vi "Acquire Image.vi"(8 "error in (no error)":errorcluster, 9 "Cluster":T2={"Gamma::Value"=1.6, "Gain::Value"=50, "Sharpness::Value"=0, "Contrast::Value"=0.5, "Exposure::Value"=0.0078125} {"Exposure::Value" min=0.000244140625 max=0.5; "Contrast::Value" min=0.0 max=1.0; "Sharpness::Value" min=0 max=2 step=1; "Gain::Value" min=0 max=100 step=1; "Gamma::Value" min=0.01 max=10.0}, 10 "Stop":bool, 11 "QR Code Reader in":refnum<class "QR Code Reader.lvclass">) -> (0 "error out":errorcluster, 2 "Image Out":T1(plugin-control), 3 "QR Code Reader out":refnum<class "QR Code Reader.lvclass">)   [LabVIEW 2021, in "QR Code Reader.lvclass"]
uses:
  QR Code Reader.lvclass
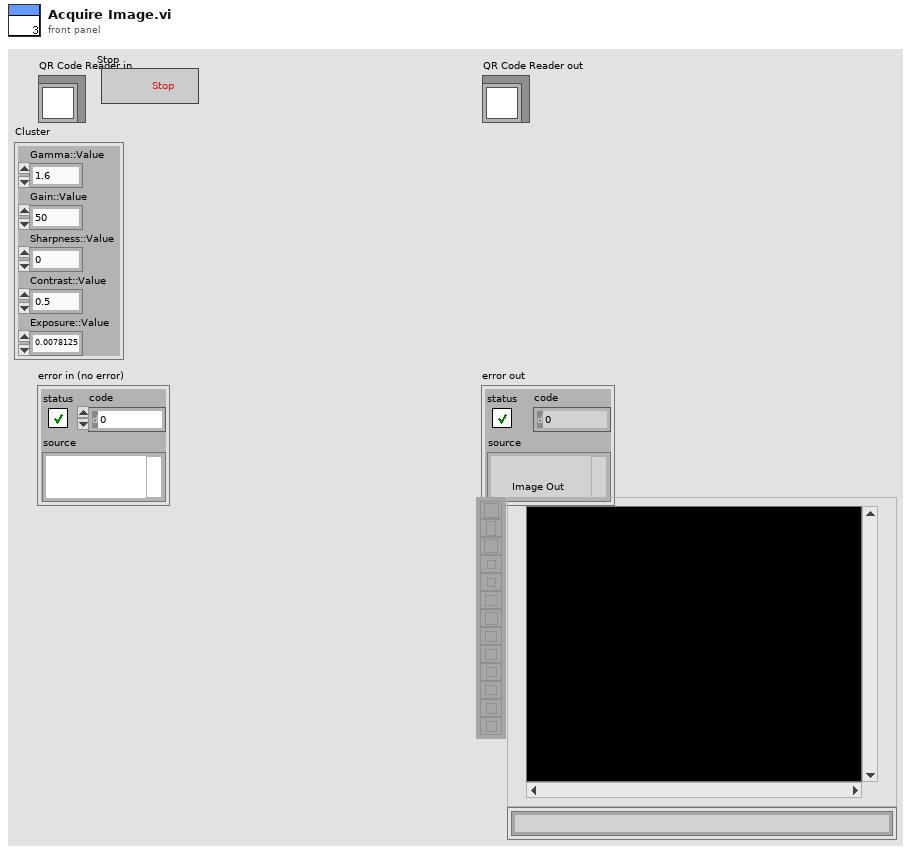
[diagram p1: front panel]
types:
  T1 = typedef "IMAQ Image.ctl" = refnum<image>
  T2 = cluster{"Gamma::Value":dbl, "Gain::Value":i64, "Sharpness::Value":i64, "Contrast::Value":dbl, "Exposure::Value":dbl}
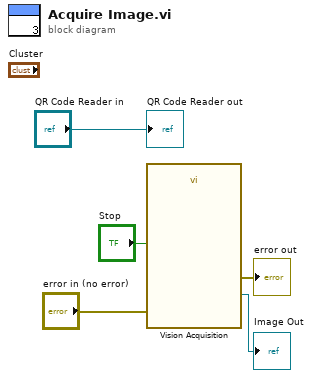
[diagram p0: block diagram]
diagram:
  n1 = call "Vision Acquisition"("Stop (F)"="Stop", "error in"="error in (no error)") -> ("Image Out"=→"Image Out":T1, "error out"=→"error out":errorcluster)  [unwired: 23 in, 1 out]
  "QR Code Reader out" <- "QR Code Reader in"
